vi "GetFile.vi"(0 "SettingsFileList in":refnum<class "SettingsFileList.lvclass">, 1 "ProjectName":string, 2 "FileName":string, 3 "MD5 (optional)":string, 5 "error in (no error)":errorcluster, 6 "Path":path) -> (14 "SettingsFileList out":refnum<class "SettingsFileList.lvclass">, 15 "BinaryData":string, 17 "HaveData":bool, 19 "error out":errorcluster)   [LabVIEW 2018, in "SettingsFileList.lvclass"]
uses:
  SettingsFileList.lvclass
  SettingsFile.lvclass
  SettingsFileList.lvclass/SettingsFileList.ctl
  SettingsFile.lvclass/SettingsFile.ctl
panel:
  out "SettingsFile out":refnum<class "SettingsFile.lvclass">
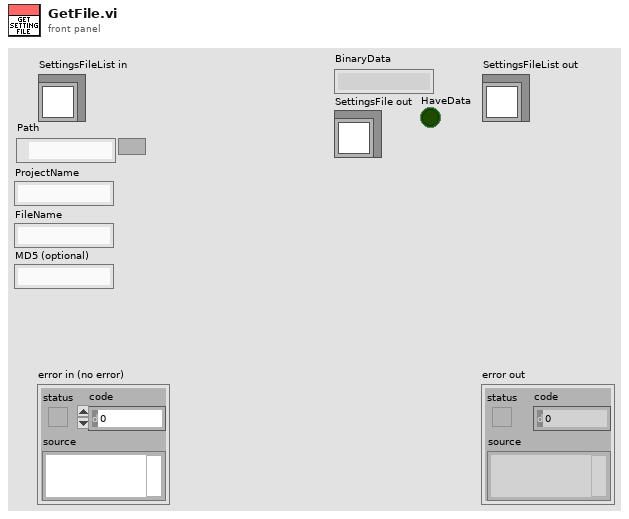
[diagram p1: front panel]
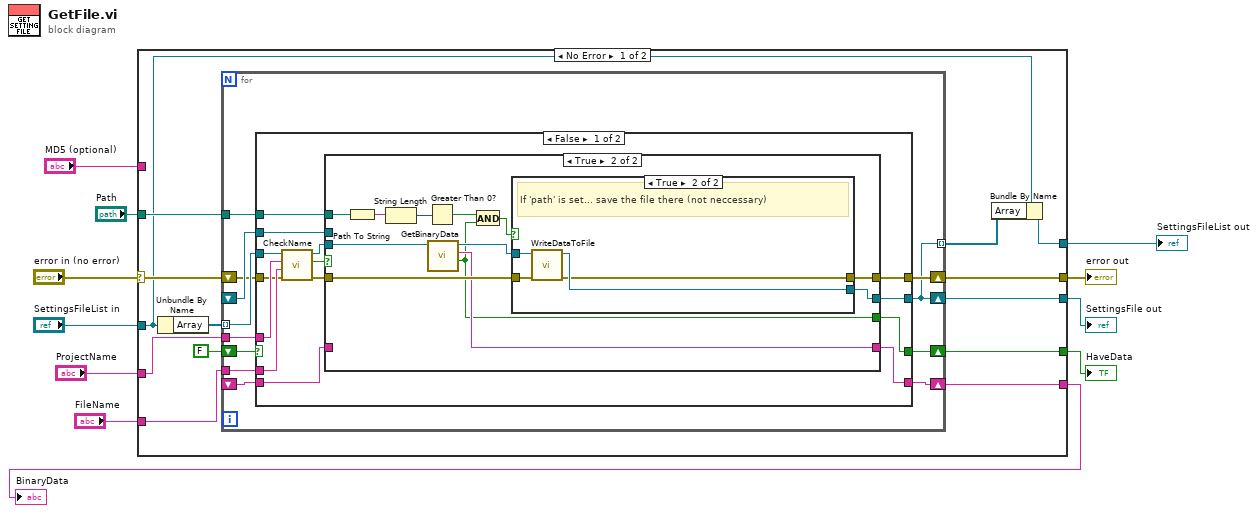
[diagram p0: block diagram]
diagram:
  n1 = case shown="No Error" "error in (no error)" {
    selector: "error in (no error)" -> [w17 w78]
    tunnel: [w16 w78] -> w10
    tunnel: [w20 _] -> w4
    tunnel: "SettingsFileList in" -> [w12 w77]
    tunnel: "Path" -> [w18 _]
    tunnel: "ProjectName" -> [w22 _]
    tunnel: "FileName" -> [w21 _]
    tunnel: "MD5 (optional)" -> [_ _]
    tunnel: [w19 _] -> w2
    tunnel: [w15 _] -> w3
    tunnel: [w13 w77] -> w1
    frame No Error {
      n2 = Unbundle By Name(w12) -> ("Array"=w24:refnum<class "SettingsFile.lvclass">[])
      n3 = for {
        tunnel: w24 -> [w36] mode=indexing
        shift-right: [w30] -> w15
        shift-left: FALSE -> [w33]
        tunnel: w22 -> [w34]
        tunnel: w21 -> [w35]
        shift-right: [w25] -> w20
        shift-left: _ -> [w32]
        shift-right: [w31] -> w19
        shift-left: _ -> [w29]
        tunnel: w18 -> [w28]
        shift-right: [w26] -> w16
        shift-left: w17 -> [w27]
        tunnel: [w25] -> w14 mode=indexing
        n4 = case shown="False" w33 {
          selector: w33 -> [_ w75]
          tunnel: w36 -> [w50 _]
          tunnel: w35 -> [w49 _]
          tunnel: w34 -> [w48 _]
          tunnel: [w46 w76] -> w25
          tunnel: w32 -> [w44 w76]
          tunnel: [w43 w74] -> w31
          tunnel: [w42 w75] -> w30
          tunnel: w29 -> [w41 w74]
          tunnel: w28 -> [w40 _]
          tunnel: w27 -> [w38 w73]
          tunnel: [w37 w73] -> w26
          frame False {
            n5 = call "CheckName.vi"("error in (no error)"=w38, "FileName"=w49, "ProjectName"=w48, "SettingsFile in"=w50) -> ("error out"=w39:errorcluster, "Boolean"=w45:bool, "SettingsFile out"=w47:refnum<class "SettingsFile.lvclass">)  [unwired: 5 in]
            n6 = case shown="True" w45 {
              selector: w45 -> [w53 _]
              tunnel: [w54 w62] -> w46
              tunnel: w47 -> [_ w60]
              tunnel: w44 -> [w54 _]
              tunnel: [w52 w56] -> w43
              tunnel: [w53 w55] -> w42
              tunnel: w41 -> [w52 _]
              tunnel: w40 -> [_ w64]
              tunnel: w39 -> [w51 w63]
              tunnel: [w51 w61] -> w37
              frame False {
              }
              frame True {
                n7 = Path To String(path=w64) -> (string=w65:string)
                n8 = String Length(string=w65) -> (length=w66:i32)
                n9 = Greater Than 0?(x=w66) -> (x > 0?=w59:bool)
                n10 = call "GetBinaryData.vi"("SettingsFile in"=w60) -> ("HaveData"=w55:bool, "BinaryData"=w56:string, "SettingsFile out"=w57:refnum<class "SettingsFile.lvclass">)  [unwired: 7 in, 1 out]
                n11 = And(x=w59, y=w55) -> (x .and. y?=w58:bool)
                n12 = case shown="True" w58 {
                  tunnel: w57 -> [w68 w72]
                  tunnel: [w68 w71] -> w62
                  tunnel: w63 -> [w67 w70]
                  tunnel: [w67 w69] -> w61
                  frame False {
                  }
                  frame True {
                    # "If 'path' is set... save the file there (not neccessary)"
                    n13 = call "WriteDataToFile.vi"("error in (no error)"=w70, "SettingsFile in"=w72) -> ("error out"=w69:errorcluster, "SettingsFile out"=w71:refnum<class "SettingsFile.lvclass">)  [unwired: 7 in, 1 out]
                  }
                }
              }
            }
          }
          frame True {
          }
        }
      }
      n14 = Bundle By Name(cluster=w12, "Array"=w14) -> (w13:refnum<class "SettingsFileList.lvclass">)
    }
    frame Error {
    }
  }
  "error out" <- w10
  "SettingsFileList out" <- w1
  "BinaryData" <- w2
  "SettingsFile out" <- w4
  "HaveData" <- w3
